vi "Day-01 pt 1 Sonar Sweep Decreasing Value Count.vi"(11 "Input":string) -> (3 "# of increases":i32)   [LabVIEW 2020, in "Advent of Code.lvlib"]
uses:
  Advent of Code.lvlib
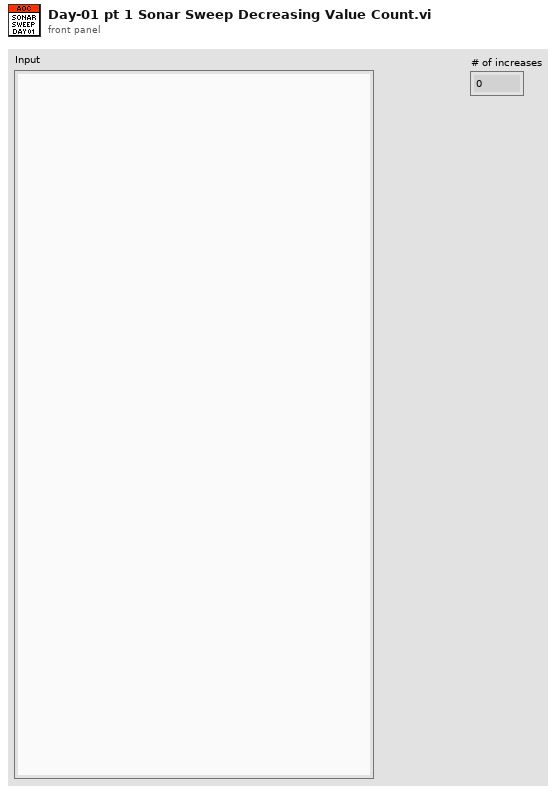
[diagram p1: front panel]
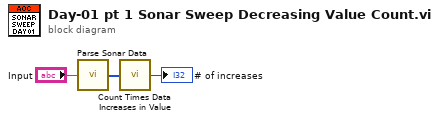
[diagram p0: block diagram]
diagram:
  n1 = call "Parse Sonar Data.vi"("Sonar Values String"="Input") -> ("Sonar Data"=w2:i32[])
  n2 = call "Count Times Data Increases in Value.vi"("Data"=w2) -> ("Count Increases"=→"# of increases":i32)
